vi "RequestFGV.vi"(7 "Actions":T1, 8 "error in (no error)":errorcluster, 9 "Data In":string, 10 "RUID":string) -> (0 "error out":errorcluster, 1 "Data Out":string)   [LabVIEW 2015]
uses:
  LVClasses/Request/Request.lvclass
  TypeDef/RequestStateCluster.ctl
  TypeDef/RequestActionEnum.ctl
panel:
  in  "Time Stamp":timestamp
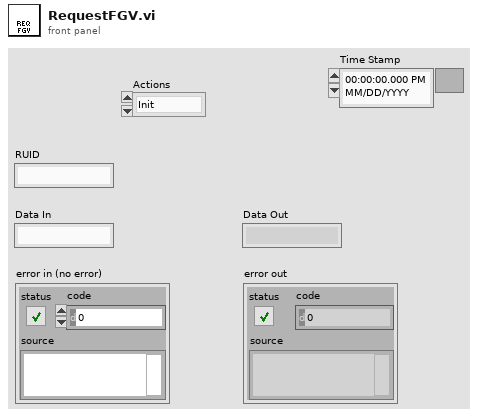
[diagram p1: front panel]
types:
  T1 = typedef "RequestActionEnum.ctl" = enum16{"Init", "ReadRequests", "ReadRequest", "AddRequest", "RemoveRequest", "ToDisk"}
  T2 = typedef "RequestStateCluster.ctl" = cluster{"Requests":refnum<class "Request.lvclass">[]}
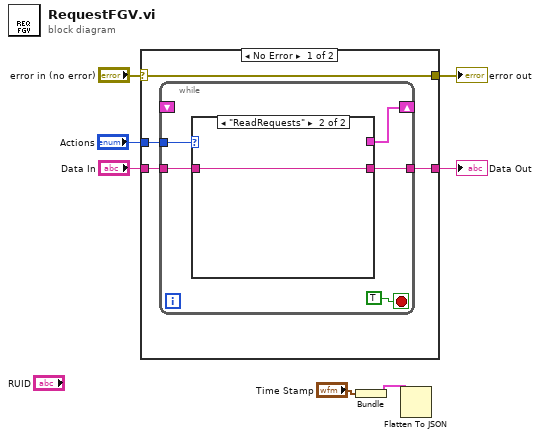
[diagram p0: block diagram]
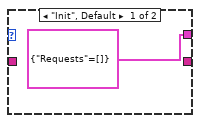
[diagram p2: hidden frame]
diagram:
  n1 = case shown="No Error" "error in (no error)" {
    selector: "error in (no error)" -> [w11 _]
    tunnel: [w11 _] -> w6
    tunnel: "Actions" -> [w10 _]
    tunnel: "Data In" -> [w9 _]
    tunnel: [w8 _] -> w3
    frame No Error {
      n2 = while {
        shift-right: [w12] -> _
        shift-left: _ -> [_]
        tunnel: w10 -> [w15]
        tunnel: w9 -> [w14]
        tunnel: [w13] -> w8
        stop <- TRUE stop-if-true
        n3 = case shown="\"ReadRequests\"" w15 {
          tunnel: w14 -> [_ w18]
          tunnel: [_ w18] -> w13
          tunnel: [T2 {"Requests"=[]} ("Cluster") _] -> w12
          frame "Init", Default {
          }
          frame "ReadRequests" {
          }
        }
      }
    }
    frame Error {
    }
  }
  "Data Out" <- w3
  "error out" <- w6
  n4 = Bundle("Time Stamp"="Time Stamp") -> (w1:cluster{"Time Stamp":timestamp})  [unwired: 1 in]
  n5 = Flatten To JSON(anything=w1) -> ()  [unwired: 2 in, 2 out]
